vi "Day 1 - Trebuchet.vi"() -> ()   [LabVIEW 2020, in "AoC 2023.lvlib"]
uses:
  AoC 2023.lvlib
panel:
  out "Puzzle Part-2 Answer":string
  out "Puzzle Answer":string
  in  "Puzzle Input":string="1abc2\npqr3stu8vwx\na1b2c3d4e5f\ntreb7uchet"
  # "Enter the Puzzle Input and run the VI"
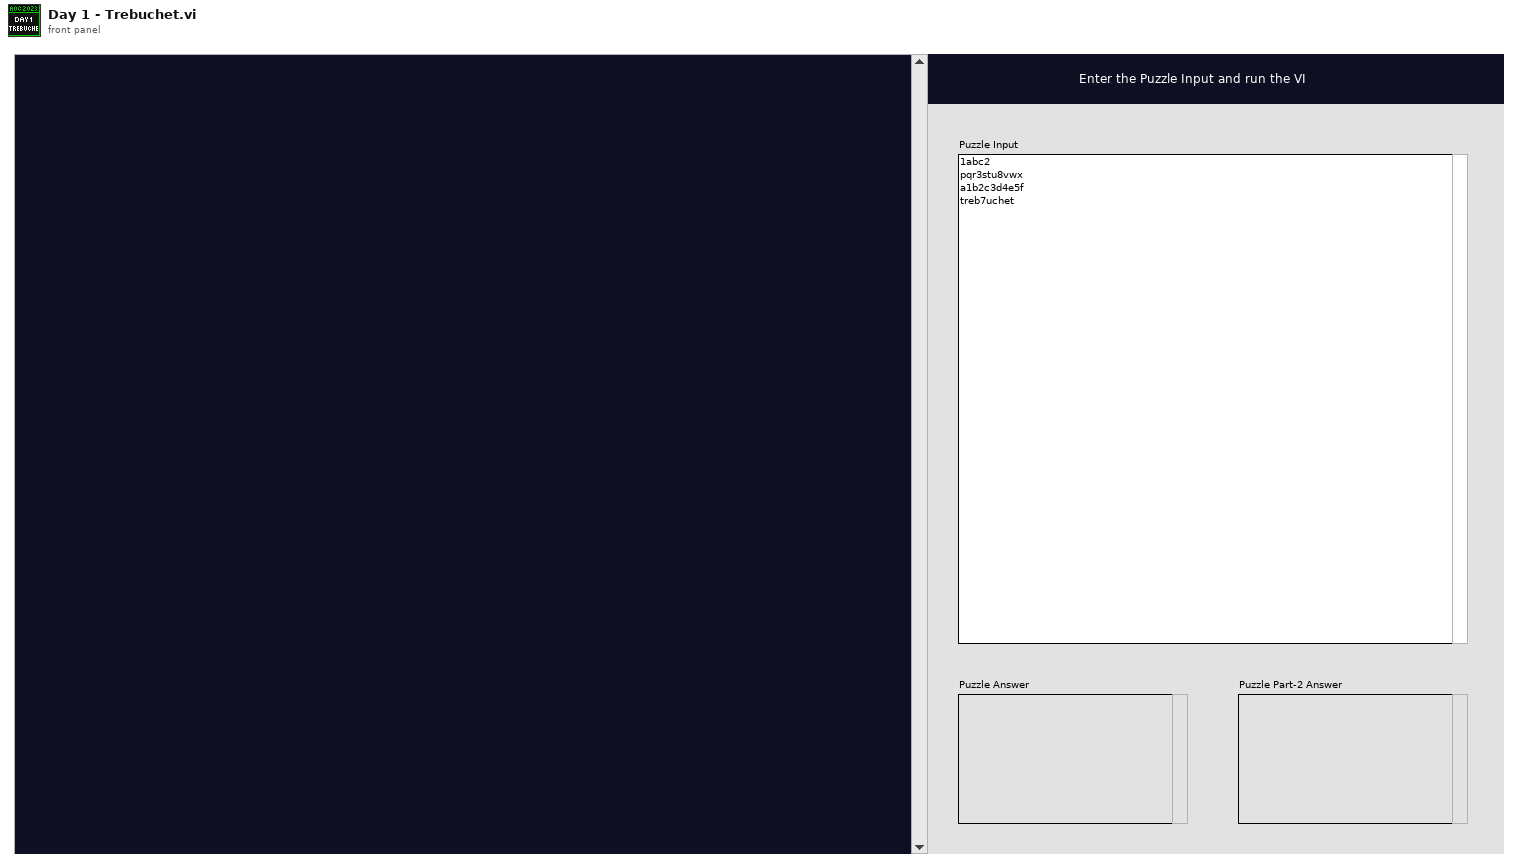
[diagram p1: front panel]
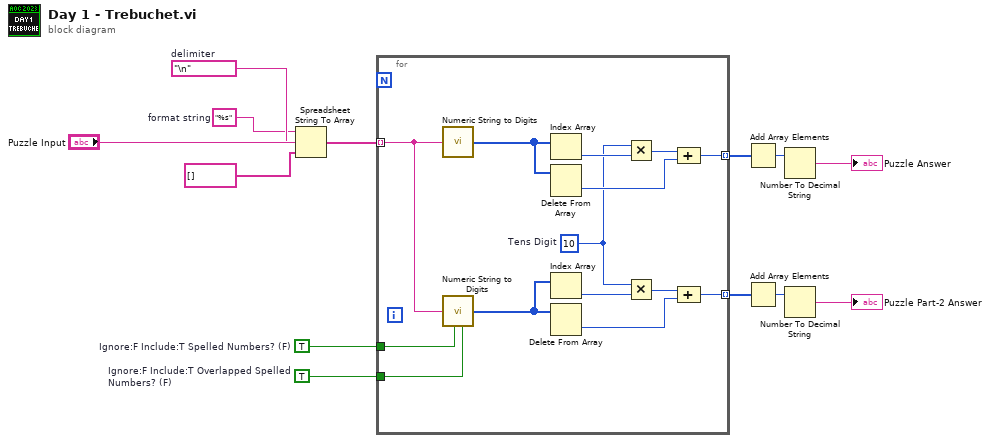
[diagram p0: block diagram]
diagram:
  w1 = TRUE  # Ignore:F Include:T Overlapped Spelled Numbers? (F)
  w6 = TRUE  # Ignore:F Include:T Spelled Numbers? (F)
  w11 = "%s"  # format string
  w12 = "\n"  # delimiter
  n1 = Spreadsheet String To Array(delimiter (Tab)=w12, format string=w11, spreadsheet string="Puzzle Input", array type (2D Dbl)=string[] []) -> (array=w9:string[])
  n2 = for {
    tunnel: w9 -> [w17] mode=indexing
    tunnel: [w26] -> w8 mode=indexing
    tunnel: w6 -> [w22]
    tunnel: [w15] -> w7 mode=indexing
    tunnel: w1 -> [w14]
    w18 = 10  # Tens Digit
    n3 = call "Numeric String to Digits.vi"("Numeric String"=w17) -> ("Digits"=w23:i32[])  [unwired: 2 in]
    n4 = call "Numeric String to Digits.vi"("Numeric String"=w17, "Ignore:F Include:T Spelled Numbers? (F)"=w22, "Ignore:F Include:T Overlapped Spelled Numbers? (F)"=w14) -> ("Digits"=w16:i32[])
    n5 = Index Array(array=w23) -> (element=w25:i32)  [unwired: 1 in]
    n6 = Delete From Array(array=w23) -> (deleted portion=w24:i32)  [unwired: 2 in, 1 out]
    n7 = Index Array(array=w16) -> (element=w20:i32)  [unwired: 1 in]
    n8 = Delete From Array(array=w16) -> (deleted portion=w21:i32)  [unwired: 2 in, 1 out]
    n9 = Multiply(x=w18, y=w25) -> (x*y=w27:i32)
    n10 = Multiply(x=w18, y=w20) -> (x*y=w19:i32)
    n11 = Compound Arithmetic op=ADD(w27, w24) -> (w26:i32)
    n12 = Compound Arithmetic op=ADD(w19, w21) -> (w15:i32)
  }
  n13 = Add Array Elements(numeric array=w8) -> (sum=w2:i32)
  n14 = Add Array Elements(numeric array=w7) -> (sum=w3:i32)
  n15 = Number To Decimal String(number=w2) -> (decimal integer string=→"Puzzle Answer":string)  [unwired: 1 in]
  n16 = Number To Decimal String(number=w3) -> (decimal integer string=→"Puzzle Part-2 Answer":string)  [unwired: 1 in]
